vi "Quasi Newton.vi"(5 "function data":T2, 7 "objective function":T3, 8 "error in (no error)":errorcluster, 9 "stopping criteria":T1={"function tolerance"=1e-06, "parameter tolerance"=1e-06, "max iterations"=100, "max function calls"=1000, "gradient tolerance"=1e-06, "max time (sec)"=-1.0}, 11 "start":dbl[](array[numeric])) -> (0 "error out":errorcluster, 1 "number of function evaluations":i32, 2 "f(minimum)":dbl, 3 "minimum":dbl[](array[numeric]))   [LabVIEW 2014, in "NI_Gmath.lvlib"]
doc: "Solves the unconstrained minimization problem for an arbitrary nonlinear function. You must manually select the polymorphic instance to use."
uses:
  NI_Gmath.lvlib
  ucno_user objective function ref.ctl
  objective function data.ctl
  stopping criteria.ctl
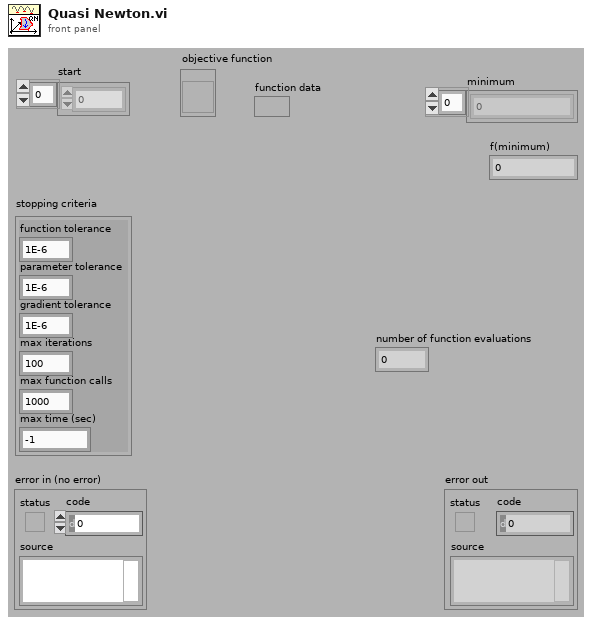
[diagram p1: front panel]
types:
  T1 = typedef "NI_Gmath.lvlib/stopping criteria.ctl" = cluster{"function tolerance":dbl, "parameter tolerance":dbl, "max iterations":i32, "max function calls":i32, "gradient tolerance":dbl, "max time (sec)":dbl}
  T2 = typedef "NI_Gmath.lvlib/objective function data.ctl" = variant
  T3 = typedef "NI_Gmath.lvlib/ucno_user objective function ref.ctl" = refnum<vi>
  T4 = cluster{"objective function":T3, "function data":T2}
  T5 = typedef "NI_Gmath.lvlib/stopping criteria with time.ctl" = cluster{"function tolerance":dbl, "parameter tolerance":dbl, "max iterations":i32, "max function calls":i32, "gradient tolerance":dbl, "max time (sec)":dbl, "initial tick count":u32}
  T6 = cluster{"objective function":bool, "gradient":bool}
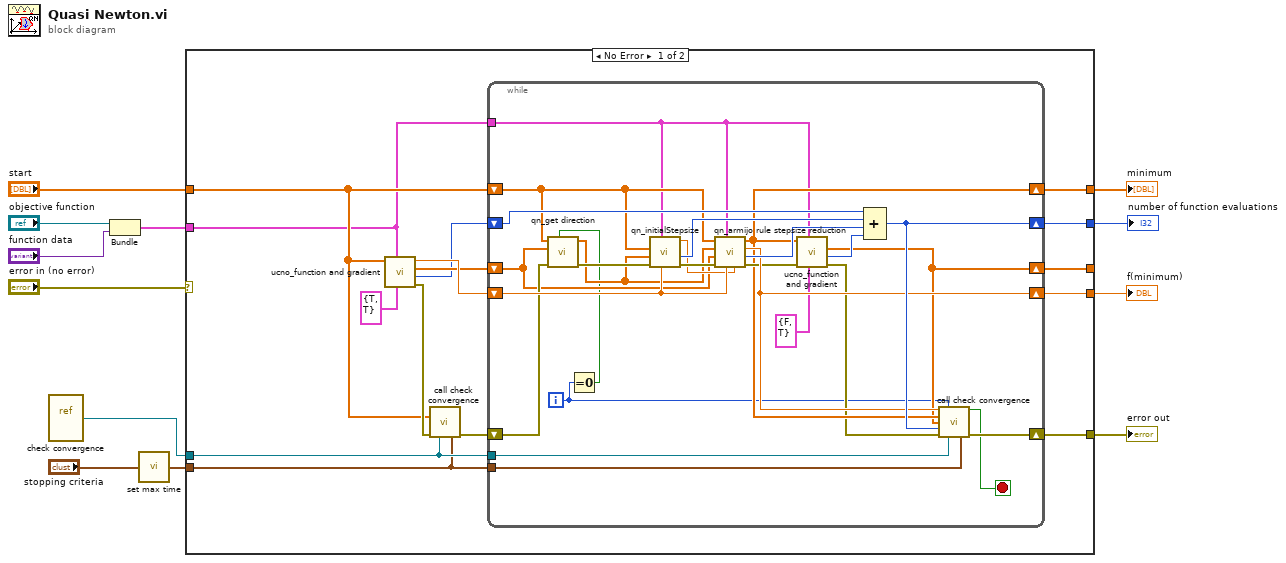
[diagram p0: block diagram]
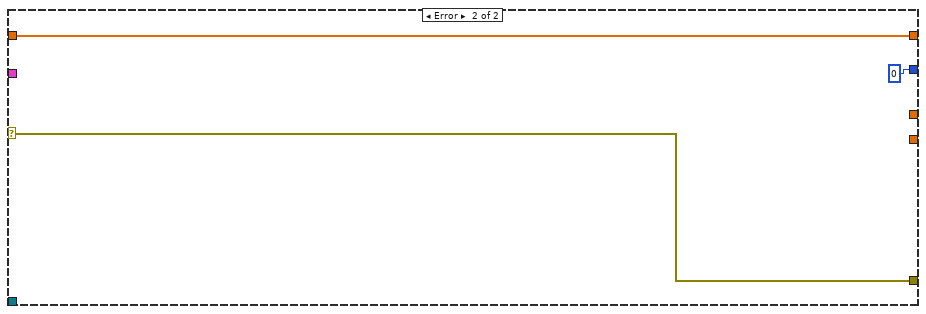
[diagram p2: hidden frame]
diagram:
  n1 = vi-ref "check convergence.vi"() -> ("vi reference"=w7:refnum<vi>)
  n2 = Bundle("objective function"="objective function", "function data"="function data") -> (w4:T4)  [unwired: 1 in]
  n3 = call "set max time.vi"("stopping criteria"="stopping criteria") -> ("stopping criteria"=w1:T5)
  n4 = case shown="No Error" "error in (no error)" {
    selector: "error in (no error)" -> [_ w56]
    tunnel: [w27 w55] -> w12
    tunnel: [w26 _] -> w11
    tunnel: [w25 _] -> _
    tunnel: "start" -> [w15 w55]
    tunnel: [w21 w56] -> w9
    tunnel: w7 -> [w24 _]
    tunnel: w1 -> [w23 _]
    tunnel: w4 -> [w13 _]
    tunnel: [w14 0 ("number of function calls")] -> w3
    frame No Error {
      n5 = call "ucno_function and gradient.vi"("output control"=T6 {"objective function"=TRUE, "gradient"=TRUE}, "function and data"=w13, "X"=w15) -> ("error out"=w17:errorcluster, "number of function calls"=w18:i32, "gradient"=w19:dbl[], "f(X)"=w20:dbl)  [unwired: 5 in]
      n6 = call "call check convergence.vi"("X"=w15, "error in"=w17, "vi reference"=w24, "stopping criteria"=w23) -> ("error out"=w22:errorcluster)  [unwired: 7 in, 4 out]
      n7 = while {
        shift-right: [w34] -> w27
        shift-left: w15 -> [w37]
        shift-right: [w33] -> w25
        shift-left: w19 -> [w36]
        tunnel: w13 -> [w31]
        shift-right: [w48] -> w26
        shift-left: w20 -> [w47]
        shift-right: [w45] -> w21
        shift-left: w22 -> [w40]
        tunnel: w24 -> [w44]
        tunnel: w23 -> [w43]
        shift-right: [w49] -> w14
        shift-left: w18 -> [w53]
        i -> [w29]
        stop <- w42 stop-if-true
        n8 = Equal To 0?(x=w29) -> (x = 0?=w28:bool)
        n9 = call "qn_get direction.vi"("reset"=w28, "error in (no error)"=w40, "gradient"=w36, "X"=w37) -> ("error out"=w39:errorcluster, "direction"=w38:dbl[])  [unwired: 6 in]
        n10 = call "qn_initialStepsize.vi"("F(X)"=w47, "function and data"=w31, "error in (no error)"=w39, "Direction"=w38, "X"=w37) -> ("error out"=w46:errorcluster, "number of function calls"=w52:i32, "s"=w41:dbl)  [unwired: 4 in]
        n11 = call "qn_armijo rule stepsize reduction.vi"("s"=w41, "F(X)"=w47, "function and data"=w31, "error in (no error)"=w46, "gradient"=w36, "Direction"=w38, "X"=w37) -> ("error out"=w35:errorcluster, "number of function calls"=w50:i32, "F(Xnew)"=w48:dbl, "Xnew"=w34:dbl[])  [unwired: 1 in]
        n12 = call "ucno_function and gradient.vi"("output control"=T6 {"objective function"=FALSE, "gradient"=TRUE}, "function and data"=w31, "error in (no error)"=w35, "X"=w34) -> ("error out"=w30:errorcluster, "number of function calls"=w51:i32, "gradient"=w33:dbl[])  [unwired: 4 in, 1 out]
        n13 = Compound Arithmetic op=ADD(w53, w52, w50, w51) -> (w49:i32)
        n14 = call "call check convergence.vi"("f"=w48, "current iteration"=w29, "X"=w34, "gradient"=w33, "number of function evaluations"=w49, "error in"=w30, "vi reference"=w44, "stopping criteria"=w43) -> ("stop?"=w42:bool, "error out"=w45:errorcluster)  [unwired: 3 in, 3 out]
      }
    }
    frame Error {
    }
  }
  "minimum" <- w12
  "f(minimum)" <- w11
  "error out" <- w9
  "number of function evaluations" <- w3
